vi "setConfigArray.vi"(8 "error in (no error)":errorcluster, 10 "ConfigArray":T1(array[cluster]), 11 "K2602 in":refnum<class "K2602.lvclass">) -> (0 "error out":errorcluster, 3 "K2602 out":refnum<class "K2602.lvclass">)   [LabVIEW 2009, in "Hardware.lvlib" / "Channels.lvlib" / "K2602.lvclass"]
uses:
  K2602.lvclass
  K2602.lvclass/K2602.ctl
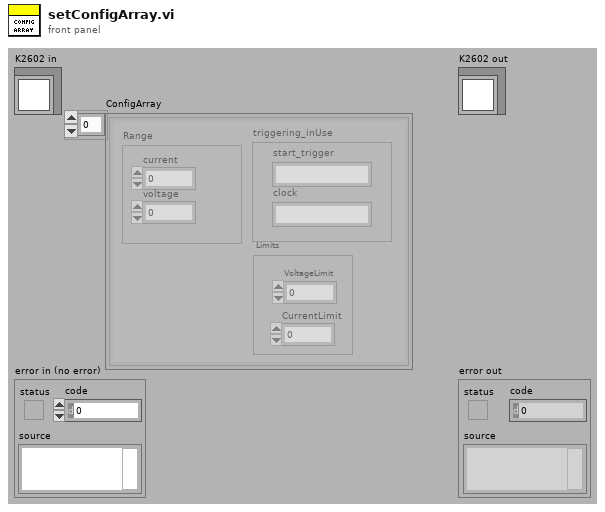
[diagram p1: front panel]
types:
  T1 = cluster{"Range":cluster{"current":dbl, "voltage":dbl}, "triggering_inUse":cluster{"start_trigger":string, "clock":string}, "Limits":cluster{"VoltageLimit":dbl, "CurrentLimit":dbl}}[]
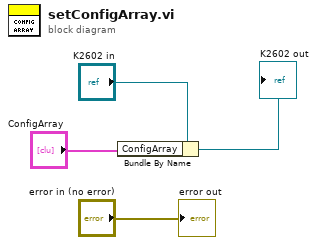
[diagram p0: block diagram]
diagram:
  n1 = Bundle By Name(cluster="K2602 in", "ConfigArray"="ConfigArray") -> (→"K2602 out":refnum<class "K2602.lvclass">)
  "error out" <- "error in (no error)"
